vi "Sync Unlock.vi"(8 "error in (no error)":errorcluster, 11 "Instrument Owner in":refnum<class "Instrument Owner.lvclass">) -> (0 "error out":errorcluster, 3 "Instrument Owner out":refnum<class "Instrument Owner.lvclass">)   [LabVIEW 2020, in "Instrument Handler.lvlib" / "Instrument Owner.lvclass"]
doc: "Release the Enqueue Lock semaphore after Instrument Msg has been fully executed."
uses:
  Instrument Owner.lvclass
  Instrument Owner.lvclass/Instrument Owner.ctl
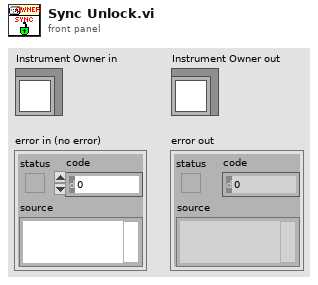
[diagram p1: front panel]
types:
  T1 = typedef "Instrument Handler.lvlib/Ctl_InstrumentSynchronicationCluster.ctl" = cluster{"Launched?":bool, "Driver Path":path, "Alias":string, "Connection Type":T2, "Pre Initialization Data":variant, "Enqueue Sync":refnum<class "Notifier.lvclass">, "Enqueue Lock":T3, "Owner Enqueuer":refnum<class "Message Enqueuer.lvclass">, "Owner":refnum<class "Sequencer Core.lvclass">, "Instrument ID":u32}
  T2 = typedef "HDH.Actor Framework.Core.Instrument Driver.lvlibp/Instrument Driver.lvclass/Ctl_ConnectionType.ctl" = enum16{"BuiltIn/System", "PXI/PCI", "USB", "GPIB", "VXI", "Serial", "TCP/IP", "cRIO", "SCXI", "cDAQ", "SwitchBlock", "SCC", "FireWire", "Accessory", "CAN", "SwitchBlock Device"}
  T3 = typedef "Semaphore RefNum" = refnum<k1>
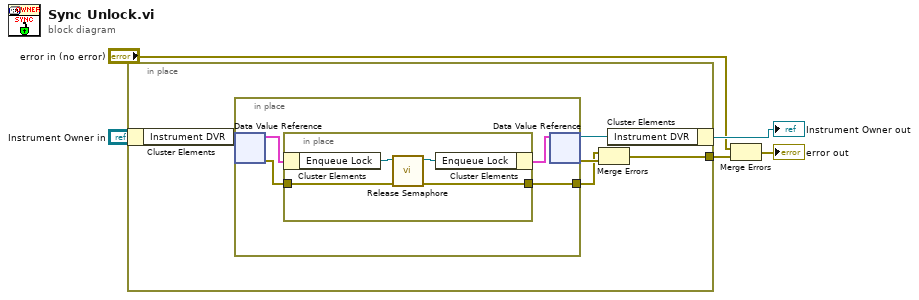
[diagram p0: block diagram]
diagram:
  n1 = in-place {
    in-place-border: [w8] -> w5
    n2 = in-place-cluster #1("Instrument Owner in") -> ("Instrument DVR"=w10:refnum<data-value>)
    n3 = in-place {
      in-place-border: [w11] -> w6
      n4 = in-place-dvr #2(w10) -> (w14:T1, w12:errorcluster)
      n5 = in-place {
        in-place-border: w12 -> [w18]
        in-place-border: [w15] -> w11
        n6 = in-place-cluster #3(w14) -> ("Enqueue Lock"=w17:T3)
        n7 = call <vilib>:"Release Semaphore.vi"("error in (no error)"=w18, "semaphore"=w17) -> ("error out"=w15:errorcluster, "semaphore out"=w16:T3)  [unwired: 4 in]
        n8 = in-place-cluster #3("Enqueue Lock"=w16) -> (w13:T1)
      }
      n9 = in-place-dvr #2(w13) -> (w9:refnum<data-value>, w7:errorcluster)
    }
    n10 = Merge Errors(w6, w7) -> (w8:errorcluster)
    n11 = in-place-cluster #1("Instrument DVR"=w9) -> (→"Instrument Owner out":refnum<class "Instrument Owner.lvclass">)
  }
  n12 = Merge Errors("error in (no error)", w5) -> (→"error out":errorcluster)
